vi "subCreateFoldersAndOpenFileForWrite.vi"(11 "File path":path) -> (0 "error out":errorcluster, 3 "File ref":refnum<file>)   [LabVIEW 2020, in "SolutionBuilder.lvlib" / "SolutionBuilder.lvclass"]
uses:
  SolutionBuilder.lvclass
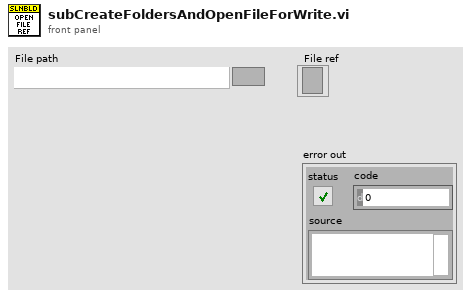
[diagram p1: front panel]
types:
  T1 = enum16{"open", "replace", "create", "open or create", "replace or create", "replace or create with confirmation"}
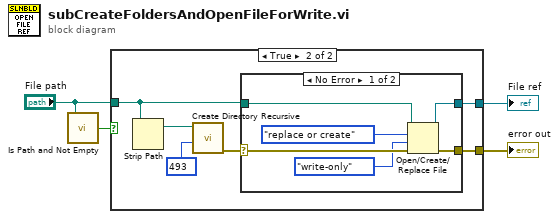
[diagram p0: block diagram]
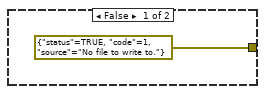
[diagram p2: hidden frame]
diagram:
  n1 = call <vilib>:"Is Path and Not Empty.vi"("path"="File path") -> ("Is Path and Not Empty?"=w4:bool)  [unwired: 4 in]
  n2 = case shown="True" w4 {
    tunnel: "File path" -> [_ w8]
    tunnel: [_ w7] -> w2
    tunnel: [errorcluster {"status"=TRUE, "code"=1, "source"="No file to write to."} ("error IO") w6] -> w1
    frame False {
    }
    frame True {
      n3 = Strip Path(path=w8) -> (stripped path=w11:path)  [unwired: 1 out]
      n4 = call <vilib>:"Create Directory Recursive.vi"("permissions"=i16 493, "directory"=w11) -> ("error out"=w9:errorcluster)  [unwired: 3 in, 2 out]
      n5 = case shown="No Error" w9 {
        selector: w9 -> [w16 w18]
        tunnel: w8 -> [w17 _]
        tunnel: [w13 _] -> w7
        tunnel: [w12 w18] -> w6
        frame No Error {
          n6 = Open/Create/Replace File(file path (use dialog)=w17, error in=w16, operation (0:open)=T1."replace or create", access (0:read/write)=enum16{"read/write", "read-only", "write-only"}."write-only") -> (refnum out=w13:refnum<file>, error out=w12:errorcluster)  [unwired: 2 in, 1 out]
        }
        frame Error {
        }
      }
    }
  }
  "File ref" <- w2
  "error out" <- w1
